vi "LM317.vi"() -> ()   [LabVIEW 2018]
panel:
  in  "V in":dbl
  in  "Potometer":dbl
  in  "R2 front":dbl
  in  "R1 front":dbl
  in  "stop":bool
  out "V out":dbl(knob) scale=-1.0..24.0
  in  "Potometer Ratio":dbl(knob) scale=0.0..100.0
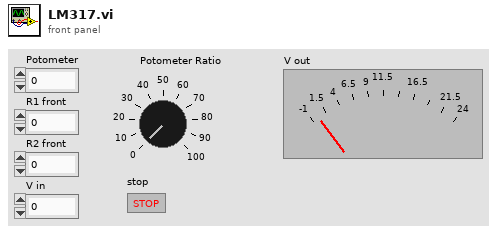
[diagram p1: front panel]
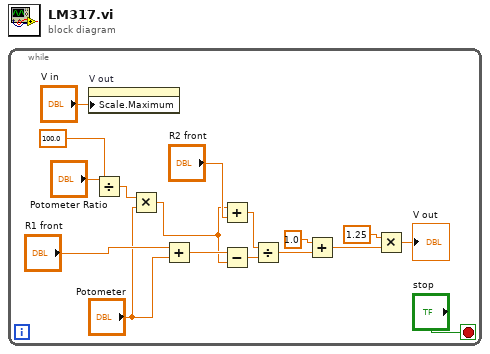
[diagram p0: block diagram]
diagram:
  n1 = while {
    stop <- "stop" stop-if-true
    n2 = property on="V out" class="Knob (strict)"("Scale.Maximum"="V in") -> ()  [unwired: 2 in, 2 out]
    n3 = Divide(x="Potometer Ratio", y=100.0) -> (x/y=w3:dbl)
    n4 = Multiply(x=w3, y="Potometer") -> (x*y=w1:dbl)
    n5 = Add(x="R1 front", y="Potometer") -> (x+y=w15:dbl)
    n6 = Add(x=w1, y="R2 front") -> (x+y=w13:dbl)
    n7 = Subtract(x=w15, y=w1) -> (x-y=w12:dbl)
    n8 = Divide(x=w13, y=w12) -> (x/y=w11:dbl)
    n9 = Add(x=1.0, y=w11) -> (x+y=w9:dbl)
    n10 = Multiply(x=1.25, y=w9) -> (x*y=→"V out":dbl)
  }
